vi "spindisk_extcontrol_init.vi"(0 "Choose Device":tag, 1 "Analog input number":i32, 3 "error in":errorcluster) -> (5 "task out":refnum<k21>, 6 "error out":errorcluster)   [LabVIEW 2016]
uses:
  <vilib>/DAQmx/create/channels.llb/DAQmx Create Channel (AI-Voltage-Basic).vi
  <resource>/objmgr/daqmx.rc
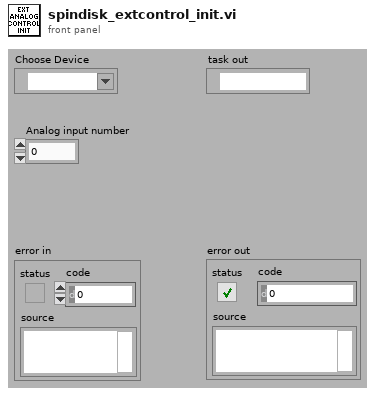
[diagram p1: front panel]
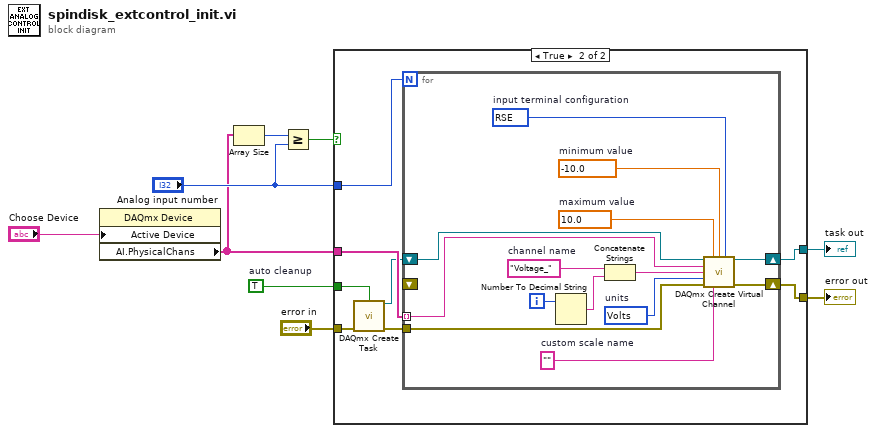
[diagram p0: block diagram]
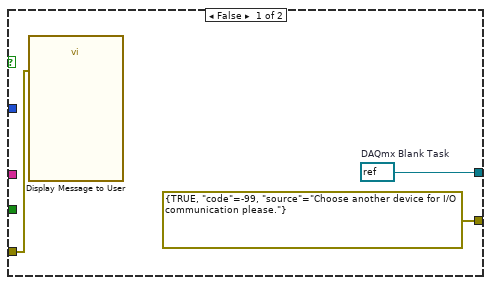
[diagram p2: hidden frame]
diagram:
  w2 = TRUE  # auto cleanup
  n1 = property class="DAQmx Device"("Active Device"="Choose Device") -> ("AI.PhysicalChans"=w6:tag[])  [unwired: 2 in, 2 out]
  n2 = Array Size(array=w6) -> (size(s)=w8:i32)
  n3 = Greater Or Equal?(x=w8, y="Analog input number") -> (x >= y?=w1:bool)
  n4 = case shown="True" w1 {
    tunnel: "error in" -> [w12 w18]
    tunnel: "Analog input number" -> [_ w20]
    tunnel: [cluster{bool, "code":i32, "source":string} {TRUE, "code"=-99, "source"="Choose another device for I/O communication please."} ("error out") w13] -> w5
    tunnel: w6 -> [_ w19]
    tunnel: [w10 w14] -> w4
    tunnel: w2 -> [_ w16]
    frame False {
      w10 = refnum<k21> refnum  # DAQmx Blank Task
      n5 = call "Display Message to User"("error in (no error)"=w12) -> ()  [unwired: 9 in, 2 out]
    }
    frame True {
      n6 = call <vilib>:"DAQmx Create Task.vi"("auto cleanup"=w16, "error in"=w18) -> ("task out"=w15:refnum<k21>, "error out"=w17:errorcluster)  [unwired: 12 in]
      n7 = for {
        N: w20 -> [_]
        tunnel: w17 -> [w34]
        tunnel: w19 -> [w23] mode=indexing
        shift-right: [w28] -> w13
        shift-left: _ -> [_]
        shift-right: [w22] -> w14
        shift-left: w15 -> [w21]
        i -> [w26]
        w29 = 10083 items=["default"=-1, "RSE"=10083, "NRSE"=10078, "Differential"=10106, "Pseudodifferential"=12529]  # input terminal configuration
        w30 = 10348 items=["Volts"=10348, "From Custom Scale"=10065]  # units
        w27 = "Voltage_"  # channel name
        w31 = ""  # custom scale name
        w32 = -10.0  # minimum value
        w33 = 10.0  # maximum value
        n8 = Number To Decimal String(number=w26) -> (decimal integer string=w25:string)  [unwired: 1 in]
        n9 = Concatenate Strings(w27, w25) -> (w24:string)
        n10 = call-poly <vilib>:"DAQmx Create Virtual Channel.vi"("task in"=w21, "maximum value"=w33, "minimum value"=w32, "input terminal configuration"=w29, "physical channels"=w23, "name to assign"=w24, "units"=w30, "error in"=w34, "custom scale name"=w31) -> ("task out"=w22:refnum<k21>, "error out"=w28:errorcluster)  [unwired: 5 in]
      }
    }
  }
  "error out" <- w5
  "task out" <- w4
